vi "Write String.vi"(8 "error in (no error)":errorcluster, 10 "String":string, 11 "String Message in":refnum<class "String Message.lvclass">) -> (0 "error out":errorcluster, 3 "String Message out":refnum<class "String Message.lvclass">)   [LabVIEW 2015, in "RDS Child Messages.lvlib" / "String Message.lvclass"]
uses:
  String Message.lvclass
  String Message.lvclass/String Message.ctl
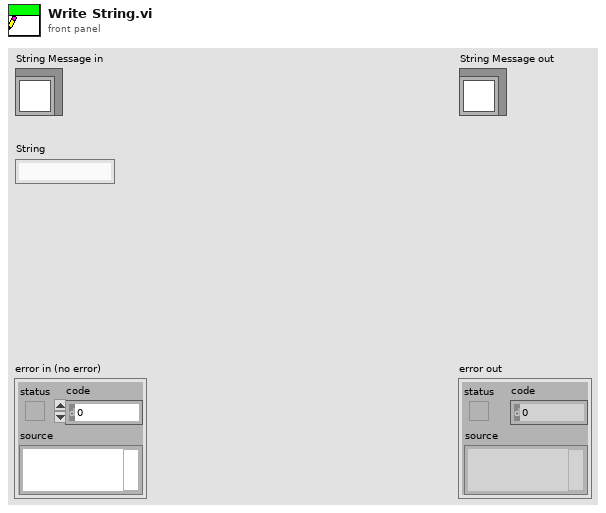
[diagram p1: front panel]
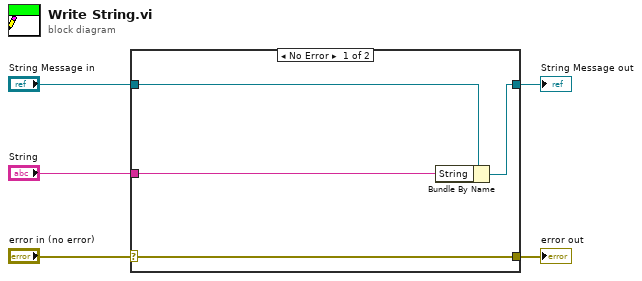
[diagram p0: block diagram]
diagram:
  n1 = case shown="No Error" "error in (no error)" {
    selector: "error in (no error)" -> [w9 w10]
    tunnel: [w9 w10] -> w4
    tunnel: [w7 w11] -> w2
    tunnel: "String Message in" -> [w8 w11]
    tunnel: "String" -> [w6 _]
    frame No Error {
      n2 = Bundle By Name(cluster=w8, "String"=w6) -> (w7:refnum<class "String Message.lvclass">)
    }
    frame Error {
    }
  }
  "error out" <- w4
  "String Message out" <- w2
